vi "Generate Draw Frame DVR.vi"(8 "Error In":errorcluster, 11 "Draw Frame In":refnum<class "Draw Frame.lvclass">) -> (0 "Error Out":errorcluster, 3 "Draw Frame Out":refnum<class "Draw Frame.lvclass">)   [LabVIEW 2019, in "Draw Frame.lvclass"]
uses:
  Draw Frame.lvclass
  Controls/Data.ctl
  <vilib>/Memosfet/myRIO-Neopixel/RT/Display/Display.lvclass
  Public/Controls/FPGA Reference.ctl
  Draw Frame.lvclass/Draw Frame.ctl
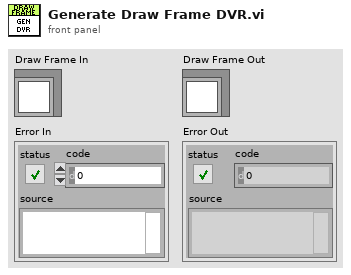
[diagram p1: front panel]
types:
  T1 = typedef "Draw Frame.lvclass/Data.ctl" = cluster{"Display":refnum<class "Display.lvclass">, "FPGA Reference":T2}
  T2 = typedef "Draw Frame.lvclass/FPGA Reference.ctl" = refnum<k20>
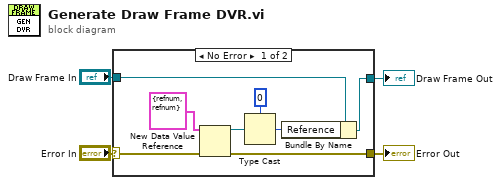
[diagram p0: block diagram]
diagram:
  n1 = case shown="No Error" "Error In" {
    selector: "Error In" -> [w12 w14]
    tunnel: "Draw Frame In" -> [w9 w13]
    tunnel: [w8 w13] -> w3
    tunnel: [w7 w14] -> w1
    frame No Error {
      n2 = New Data Value Reference(data value=T1 {"Display"=refnum, "FPGA Reference"=refnum} ("Data"), error in=w12) -> (data value reference=w11:refnum<data-value>, error out=w7:errorcluster)
      n3 = Type Cast(type=u64 0, x=w11) -> (*(type *) &x=w6:u64)
      n4 = Bundle By Name(cluster=w9, "Reference"=w6) -> (w8:refnum<class "Draw Frame.lvclass">)
    }
    frame Error {
    }
  }
  "Error Out" <- w1
  "Draw Frame Out" <- w3
